vi "运维调试_其他.vi"() -> ()   [LabVIEW 2016, in "其他.lvlib"]
uses:
  <vilib>/Utility/miscctls.llb/LVPointTypeDef.ctl
  PLC/PLC.lvlib
panel:
  out "集成报警信息":string
  out "R115":i16 caption="灯带关闭时间"
  out "R114":i16 caption="灯带开启时间"
  in  "视频监控":bool
  in  "照明":bool
  in  "前门灯带":bool
  in  "侧边灯带":bool
  in  "返回":bool
  in  "设置":bool
  # "参数设置"
  # "H"
  # "H"
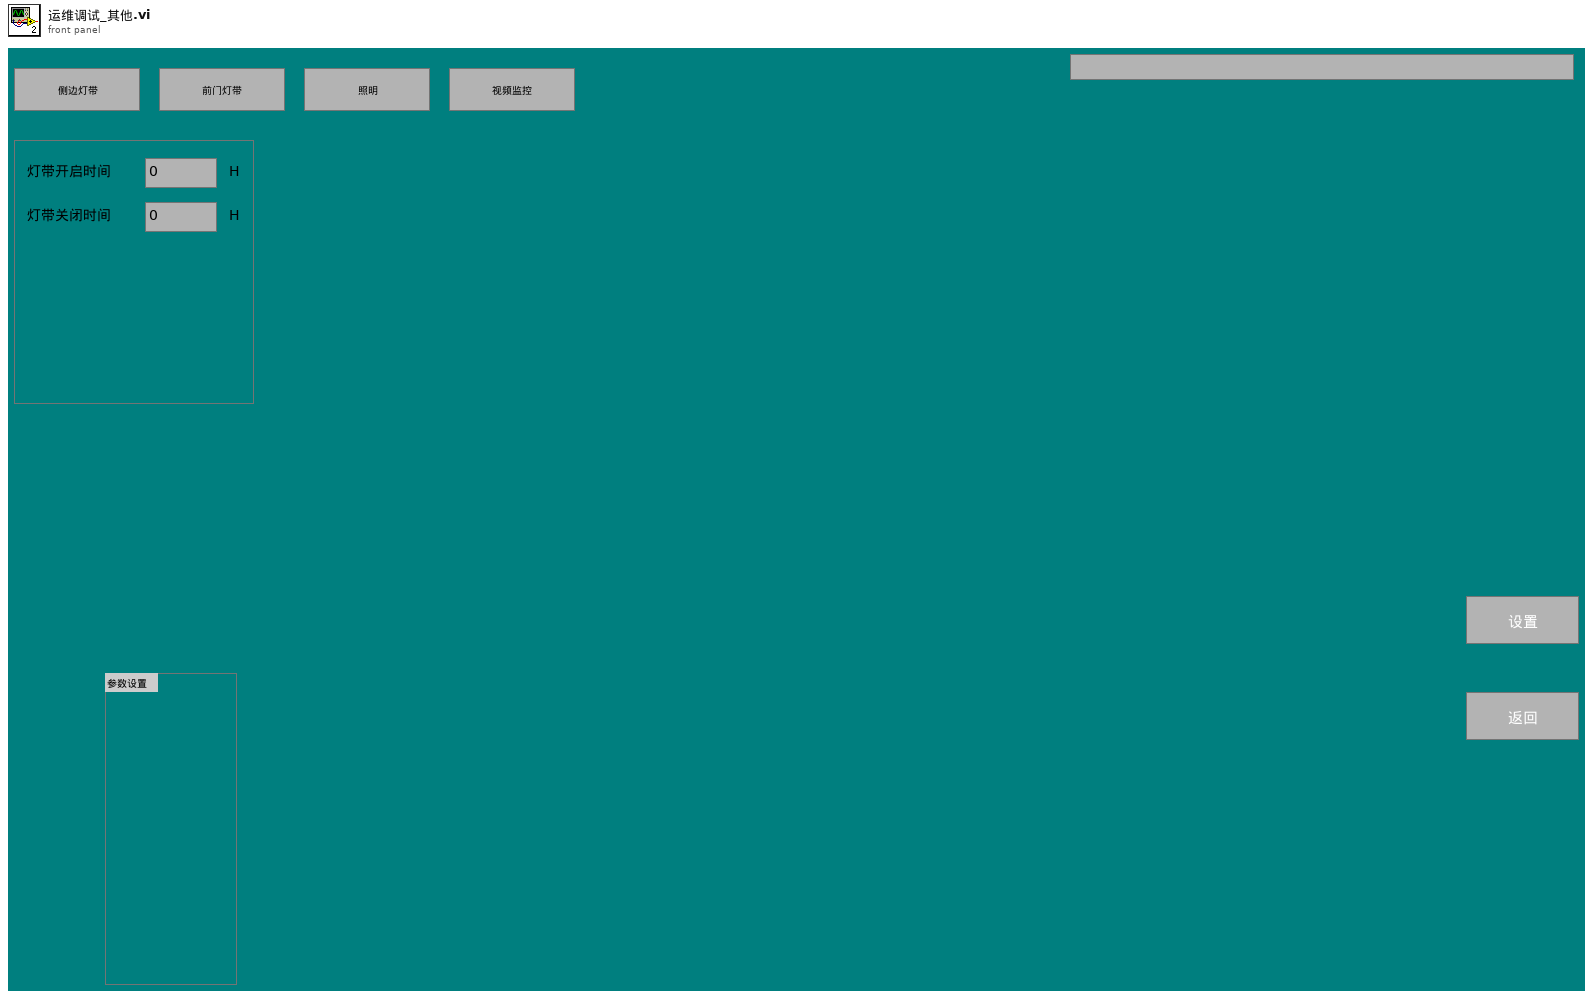
[diagram p1: front panel]
types:
  T1 = cluster{"R100":i16, "R101":i16, "R102":i16, "R103":i16, "R104":i16, "R105":i16, "R106":i16, "R107":i16, "R108":i16, "R109":i16, "R110":i16, "R111":i16, "R112":i16, "R113":i16, "R114":i16, "R115":i16, "R116":i16, "R117":i16, "R118":i16, "R119":i16}
  T2 = cluster{"Y0":bool, "Y1":bool, "Y2":bool, "Y3":bool, "Y4":bool, "Y5":bool, "Y6":bool, "Y7":bool, "Y8":bool, "Y9":bool, "Y10":bool, "Y11":bool, "Y12":bool, "Y13":bool, "Y14":bool, "Y15":bool}
  T3 = cluster{"coil values[0]":bool, "coil values[1]":bool, "coil values[2]":bool, "coil values[3]":bool, "coil values[4]":bool, "coil values[5]":bool, "coil values[6]":bool, "coil values[7]":bool, "coil values[8]":bool, "coil values[9]":bool, "coil values[10]":bool, "coil values[11]":bool, "coil values[12]":bool, "coil values[13]":bool, "coil values[14]":bool, "coil values[15]":bool}
  T4 = typedef "LVPointTypeDef.ctl" = cluster{"Horizontal":i16, "Vertical":i16}
  T5 = cluster{"命令":string, "data":cluster{"starting address":u16, "coil values":bool[]}}
  T6 = cluster{"命令":string, "数据":cluster{"starting address":u16, "holding register values":u16[]}}
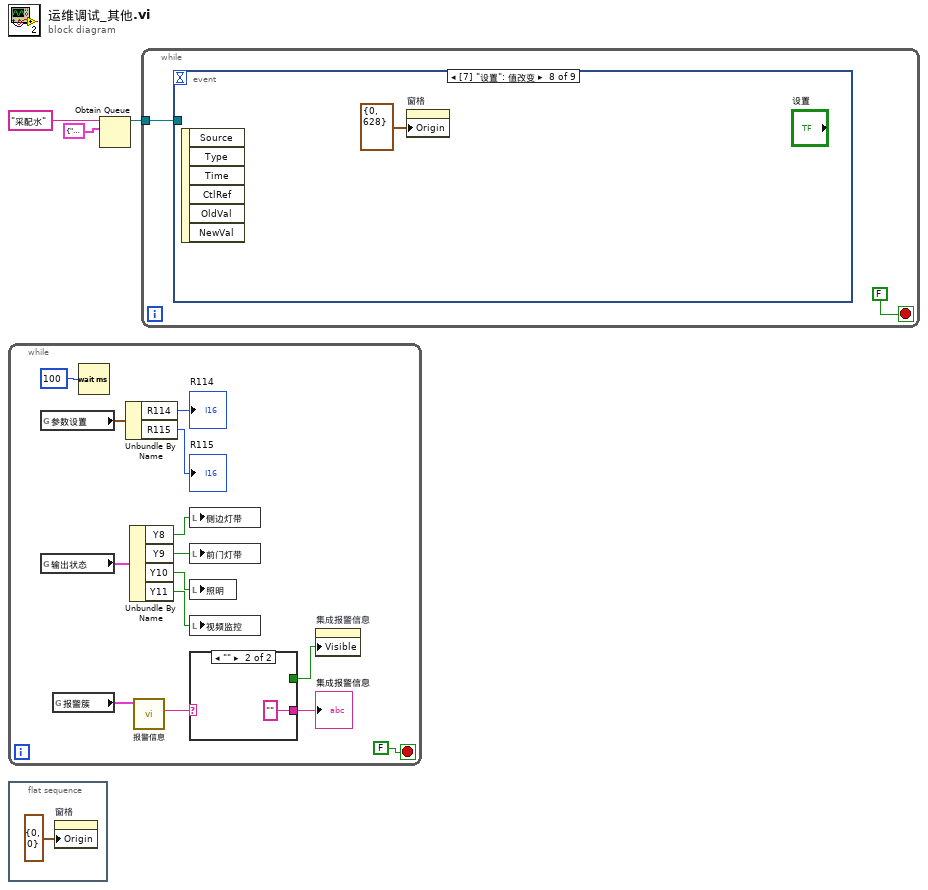
[diagram p0: block diagram]
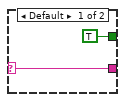
[diagram p2: hidden frame]
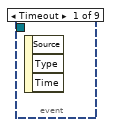
[diagram p3: hidden frame]
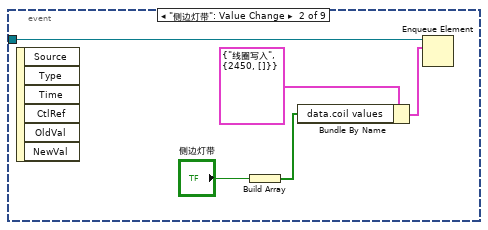
[diagram p4: hidden frame]
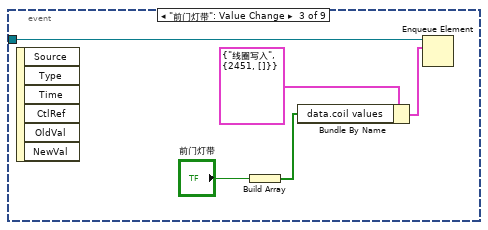
[diagram p5: hidden frame]
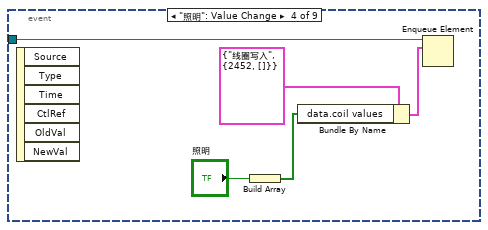
[diagram p6: hidden frame]
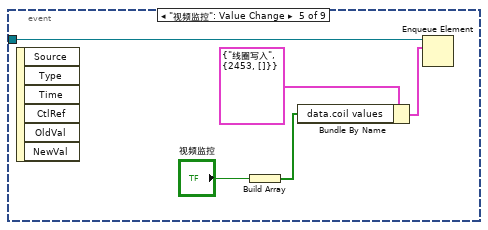
[diagram p7: hidden frame]
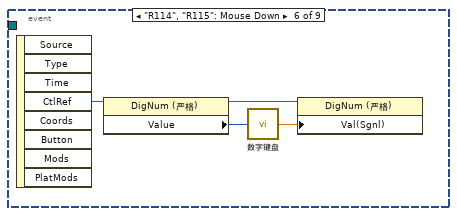
[diagram p8: hidden frame]
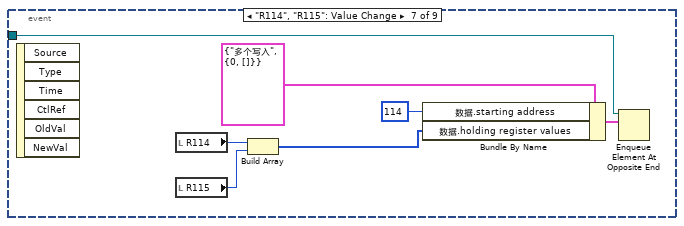
[diagram p9: hidden frame]
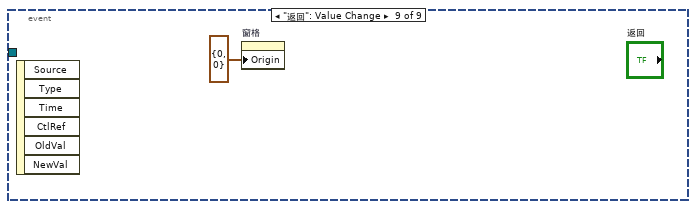
[diagram p10: hidden frame]
diagram:
  n1 = while {
    stop <- FALSE stop-if-true
    n2 = global read "采配水全局变量.vi" "参数设置"() -> (w14:T1)
    n3 = global read "采配水全局变量.vi" "输出状态"() -> (w15:T2)
    n4 = global read "采配水全局变量.vi" "报警簇"() -> (w8:T3)
    n5 = Wait (ms)(milliseconds to wait=u32 100 ("等待时间（毫秒）")) -> ()  [unwired: 1 out]
    n6 = Unbundle By Name(w14) -> ("R114"=→"R114":i16, "R115"=→"R115":i16)
    n7 = Unbundle By Name(w15) -> ("Y8"=w7:bool, "Y9"=w6:bool, "Y10"=w5:bool, "Y11"=w4:bool)
    n8 = call "报警信息.vi"("报警簇"=w8) -> ("系统报警信息"=w11:string)  [unwired: 9 in, 1 out]
    n9 = local write "侧边灯带"(w7) -> ()
    n10 = local write "前门灯带"(w6) -> ()
    n11 = local write "照明"(w5) -> ()
    n12 = local write "视频监控"(w4) -> ()
    n13 = case shown="\"\"" w11 {
      selector: w11 -> [w19 _]
      tunnel: [w19 "" ("字符串")] -> w9
      tunnel: [TRUE ("可见") _] -> w10
      frame Default {
      }
      frame "" {
      }
    }
    "集成报警信息" <- w9
    n14 = property on="集成报警信息" class="Str"("Visible"=w10) -> ()  [unwired: 2 in, 2 out]
  }
  n15 = flat-sequence {
    frame #0 {
      n16 = property on="窗格" class="Pane"("Origin"=T4 {"Horizontal"=0, "Vertical"=0} ("原点")) -> ()  [unwired: 2 in, 2 out]
    }
  }
  n17 = Obtain Queue(name (unnamed)="采配水" ("名称（未命名）"), element data type=cluster{"命令":string, "数据":variant} {"命令"="", "数据"=variant}) -> (queue out=w1:refnum<queue>)  [unwired: 3 in, 2 out]
  n18 = while {
    tunnel: w1 -> [w22]
    stop <- FALSE stop-if-true
    n19 = event shown="[7] \"设置\": 值改变" {
      selector: _ -> [_ _ _ _ _ _ _ _ _]
      dyn-events: _ -> [_ _ _ _ _ _ _ _ _]
      timeout: _ -> [_ _ _ _ _ _ _ _ _]
      tunnel: w22 -> [_ w25 w31 w36 w41 _ w48 _ _]
      event Timeout {
        n20 = event-data() -> ()  [unwired: 1 in, 3 out]
      }
      event "侧边灯带": Value Change {
        n21 = event-data() -> ()  [unwired: 1 in, 6 out]
        n22 = Build Array("侧边灯带") -> (w24:bool[])
        n23 = Bundle By Name(cluster=T5 {"命令"="线圈写入", "data"={"starting address"=2450, "coil values"=[]}} ("元素"), "data.coil values"=w24) -> (w26:T5)
        n24 = Enqueue Element(queue=w25, element=w26) -> ()  [unwired: 2 in, 3 out]
      }
      event "前门灯带": Value Change {
        n25 = event-data() -> ()  [unwired: 1 in, 6 out]
        n26 = Build Array("前门灯带") -> (w30:bool[])
        n27 = Bundle By Name(cluster=T5 {"命令"="线圈写入", "data"={"starting address"=2451, "coil values"=[]}} ("元素"), "data.coil values"=w30) -> (w32:T5)
        n28 = Enqueue Element(queue=w31, element=w32) -> ()  [unwired: 2 in, 3 out]
      }
      event "照明": Value Change {
        n29 = event-data() -> ()  [unwired: 1 in, 6 out]
        n30 = Build Array("照明") -> (w35:bool[])
        n31 = Bundle By Name(cluster=T5 {"命令"="线圈写入", "data"={"starting address"=2452, "coil values"=[]}} ("元素"), "data.coil values"=w35) -> (w37:T5)
        n32 = Enqueue Element(queue=w36, element=w37) -> ()  [unwired: 2 in, 3 out]
      }
      event "视频监控": Value Change {
        n33 = event-data() -> ()  [unwired: 1 in, 6 out]
        n34 = Build Array("视频监控") -> (w40:bool[])
        n35 = Bundle By Name(cluster=T5 {"命令"="线圈写入", "data"={"starting address"=2453, "coil values"=[]}} ("元素"), "data.coil values"=w40) -> (w42:T5)
        n36 = Enqueue Element(queue=w41, element=w42) -> ()  [unwired: 2 in, 3 out]
      }
      event "R114", "R115": Mouse Down {
        n37 = event-data() -> ("CtlRef"=w47:refnum<vi>)  [unwired: 1 in, 7 out]
        n38 = property class="DigNum (严格)"(reference=w47) -> (reference out=w46:refnum<vi>, "Value"=w45:i16)  [unwired: 1 in, 1 out]
        n39 = call "数字键盘.vi"("OldNumber"=w45) -> ("NewNumber"=w44:sgl)
        n40 = property class="DigNum (严格)"(reference=w46, "Val(Sgnl)"=w44) -> ()  [unwired: 1 in, 2 out]
      }
      event "R114", "R115": Value Change {
        n41 = event-data() -> ()  [unwired: 1 in, 6 out]
        n42 = local read "R114"() -> (w53:i16)
        n43 = local read "R115"() -> (w54:i16)
        n44 = Build Array(w53, w54) -> (w49:i16[])
        n45 = Bundle By Name(cluster=T6 {"命令"="多个写入", "数据"={"starting address"=0, "holding register values"=[]}} ("元素"), "数据.starting address"=u16 114, "数据.holding register values"=w49) -> (w50:T6)
        n46 = Enqueue Element At Opposite End(queue=w48, element=w50) -> ()  [unwired: 2 in, 3 out]
      }
      event "设置": Value Change {
        n47 = event-data() -> ()  [unwired: 1 in, 6 out]
        n48 = property on="窗格" class="Pane"("Origin"=T4 {"Horizontal"=0, "Vertical"=628} ("原点")) -> ()  [unwired: 2 in, 2 out]
      }
      event "返回": Value Change {
        n49 = event-data() -> ()  [unwired: 1 in, 6 out]
        n50 = property on="窗格" class="Pane"("Origin"=T4 {"Horizontal"=0, "Vertical"=0} ("原点")) -> ()  [unwired: 2 in, 2 out]
      }
    }
  }
